vi "Pre Launch Init.vi"(11 "CoordinatorState in":refnum<class "CoordinatorState.lvclass"> caption="操作者输入") -> (0 "error out":errorcluster caption="错误输出", 3 "CoordinatorState out":refnum<class "CoordinatorState.lvclass"> caption="操作者输出")   [LabVIEW 2014, in "States.lvlib" / "CoordinatorState.lvclass"]
doc: "(<B>Filename</B>: Actor Framework.lvlib:Actor.lvclass:Pre Launch Init.vi)\n\nDefines behavior that occurs after the Launch Nested Actor method is invoked but before the actor's Actor Core method begins running.\n\nBy default, this method does nothing. A descendant class may override it to define behavior."
uses:
  CoordinatorState.lvclass
  CoordinatorState.lvclass/CoordinatorState.ctl
  <vilib>/NI/Actors/State Actor/State Actor/State Actor.lvclass
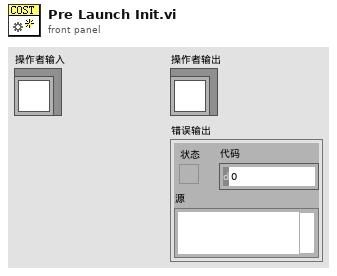
[diagram p1: front panel]
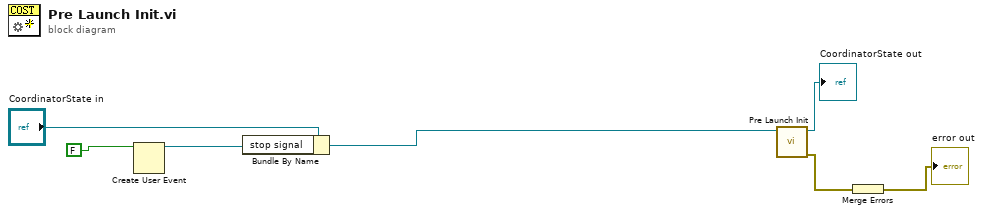
[diagram p0: block diagram]
diagram:
  n1 = Create User Event(user event datatype=FALSE ("stop signal")) -> (user event=w4:refnum<user-event>)  [unwired: 1 in, 1 out]
  n2 = Bundle By Name(cluster="CoordinatorState in", "stop signal"=w4) -> (w1:refnum<class "CoordinatorState.lvclass">)
  n3 = call-parent "Pre Launch Init.vi"("Actor in"=w1) -> ("error out"=w6:errorcluster, "Actor out"=→"CoordinatorState out":refnum<class "CoordinatorState.lvclass">)  [unwired: 9 in]
  n4 = Merge Errors(w6) -> (→"error out":errorcluster)
